vi "Str to Conn Cluster.vi"(0 "Str":string) -> (6 "Conn str":T1)   [LabVIEW 2014]
uses:
  Ctr/Constr.ctl
  <vilib>/addons/database/Connection.llb/Conn ObjectReference.ctl
  <vilib>/addons/database/NI_Database_API.lvlib
  Ctr/Conneect State.ctl
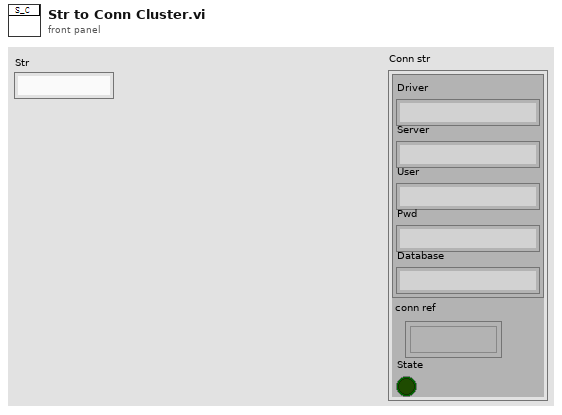
[diagram p1: front panel]
types:
  T1 = typedef "Conneect State.ctl" = cluster{"Constr":T2, "conn ref":T3, "State":bool}
  T2 = typedef "Constr.ctl" = cluster{"Driver":string, "Server":string, "User":string, "Pwd":string, "Database":string}
  T3 = typedef "NI_Database_API.lvlib/Conn ObjectReference.ctl" = refnum<k1>
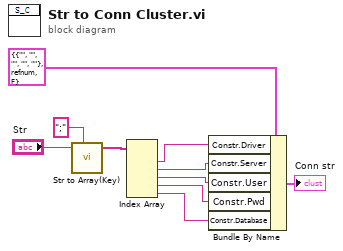
[diagram p0: block diagram]
diagram:
  n1 = call "Str to Array(Key).vi"("Str"="Str", "Key"=";") -> ("Str Array"=w7:string[])  [unwired: 7 in]
  n2 = Index Array(array=w7) -> (element #1=w6:string, element #2=w5:string, element #3=w4:string, element #4=w3:string, element #5=w2:string)  [unwired: 5 in]
  n3 = Bundle By Name(cluster=T1 {"Constr"={"Driver"="", "Server"="", "User"="", "Pwd"="", "Database"=""}, "conn ref"=refnum, "State"=FALSE} ("Connncet State"), "Constr.Driver"=w6, "Constr.Server"=w5, "Constr.User"=w4, "Constr.Pwd"=w3, "Constr.Database"=w2) -> (→"Conn str":T1)
